vi "Get Local Color Table.vi"(8 "error in (no error)":errorcluster caption="错误输入（无错误）", 9 "Image Descriptor":T1, 11 "Gif Image 输入":refnum<class "Gif Image.lvclass"> caption="DNL_LabVIEW Object in") -> (0 "error out":errorcluster caption="错误输出", 1 "Color Table":u32[](array[numeric]), 3 "Gif Image 输出":refnum<class "Gif Image.lvclass"> caption="DNL_LabVIEW Object out")   [LabVIEW 2011, in "Gif Image.lvclass"]
uses:
  Gif Image.lvclass
  Control/Image Descriptor.ctl
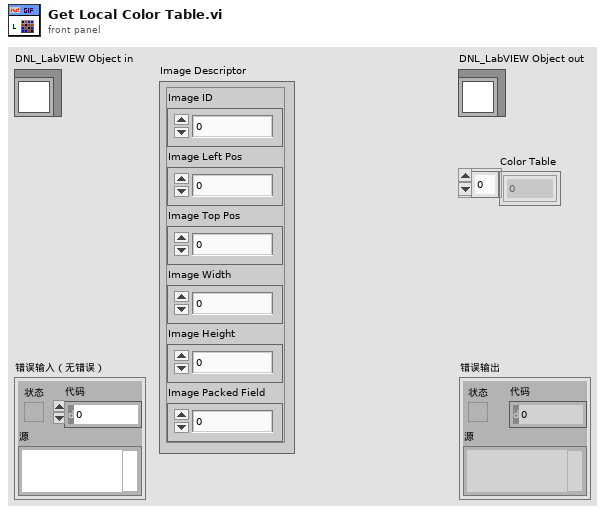
[diagram p1: front panel]
types:
  T1 = typedef "Gif Image.lvclass/Image Descriptor.ctl" = cluster{"Image ID":u8, "Image Left Pos":u16, "Image Top Pos":u16, "Image Width":u16, "Image Height":u16, "Image Packed Field":u8}
  T2 = typedef "Gif Image.lvclass/Image Packed Field.ctl" = cluster{"Local Color Table Flag ":bool, "Interlace Flag":bool, "Sort Flag":bool, "Reserved":u8, "Size of Color Table":u8}
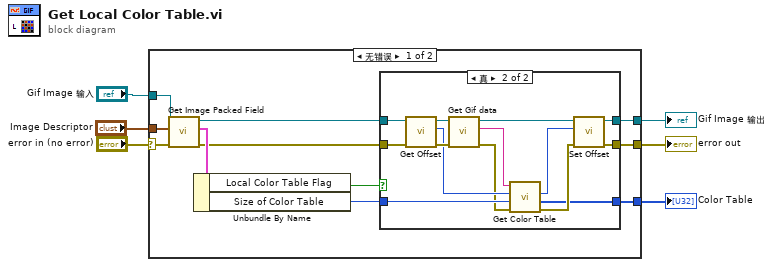
[diagram p0: block diagram]
diagram:
  n1 = case shown="无错误" "error in (no error)" {
    selector: "error in (no error)" -> [w15 w35]
    tunnel: [w7 w35] -> w5
    tunnel: [w8 w34] -> w3
    tunnel: "Gif Image 输入" -> [w17 w34]
    tunnel: "Image Descriptor" -> [w16 _]
    tunnel: [w9 _] -> w1
    frame No Error {
      n2 = call "Get Image Packed Field.vi"("error in (no error)"=w15, "Image Descriptor"=w16, "Gif Image 输入"=w17) -> ("error out"=w12:errorcluster, "Image Packed Filed"=w14:T2, "Gif Image 输出"=w13:refnum<class "Gif Image.lvclass">)  [unwired: 6 in]
      n3 = Unbundle By Name(w14) -> ("Local Color Table Flag"=w10:bool, "Size of Color Table"=w11:u8)
      n4 = case shown="真" w10 {
        tunnel: w13 -> [w19 w33]
        tunnel: w12 -> [w18 w31]
        tunnel: w11 -> [_ w27]
        tunnel: [_ w22] -> w9
        tunnel: [w19 w21] -> w8
        tunnel: [w18 w20] -> w7
        frame False {
        }
        frame True {
          n5 = call "Get Offset.vi"("error in (no error)"=w31, "Gif Image输入"=w33) -> ("error out"=w30:errorcluster, "Offset"=w29:i32, "Gif Image输出"=w32:refnum<class "Gif Image.lvclass">)  [unwired: 7 in]
          n6 = call "Get Gif data.vi"("error in (no error)"=w30, "Gif Image输入"=w32) -> ("error out"=w26:errorcluster, "Gif data"=w28:string, "Gif Image输出"=w24:refnum<class "Gif Image.lvclass">)  [unwired: 7 in]
          n7 = call "Get Color Table.vi"("错误输入"=w26, "Size of Color Table"=w27, "Offset In"=w29, "Gif data In"=w28) -> ("错误输出"=w23:errorcluster, "Color Table"=w22:u32[], "Offset Out"=w25:i32)  [unwired: 4 in, 1 out]
          n8 = call "Set Offset.vi"("error in (no error)"=w23, "Offset"=w25, "Gif Image输入"=w24) -> ("error out"=w20:errorcluster, "Gif Image输出"=w21:refnum<class "Gif Image.lvclass">)  [unwired: 7 in]
        }
      }
    }
    frame Error {
    }
  }
  "error out" <- w5
  "Gif Image 输出" <- w3
  "Color Table" <- w1
